vi "temp_calc.vi"(10 "[C/K]":bool, 11 "T (F)":dbl) -> (3 "Out temp [C/K]":dbl)   [LabVIEW 2017]
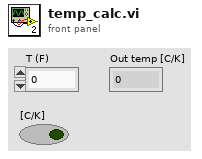
[diagram p1: front panel]
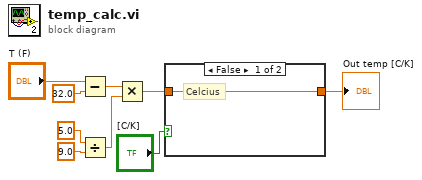
[diagram p0: block diagram]
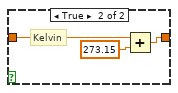
[diagram p2: hidden frame]
diagram:
  n1 = Subtract(x="T (F)", y=32.0) -> (x-y=w6:dbl)
  n2 = Divide(x=5.0, y=9.0) -> (x/y=w7:dbl)
  n3 = Multiply(x=w6, y=w7) -> (x*y=w8:dbl)
  n4 = case shown="False" "[C/K]" {
    tunnel: w8 -> [w10 w13]
    tunnel: [w10 w11] -> w9
    frame False {
      # "Celcius"
    }
    frame True {
      # "Kelvin"
      n5 = Add(x=w13, y=273.15) -> (x+y=w11:dbl)
    }
  }
  "Out temp [C/K]" <- w9
